vi "getWavelength_v80AM.vi"() -> ()   [LabVIEW 2016]
uses:
  x32/CLDevIFace.dll
panel:
  in  "Delay Time (s)":dbl=0.01
  out "XY Graph":cluster{i32[], dbl[]}(graph)
  out "error out":errorcluster
  out "output param":i32
  in  "stop":bool
  in  "OK Button":bool
  out "Wavelength":dbl format="%.9f"
  in  "CommPort":dbl=5.0 caption="Comm Port #"
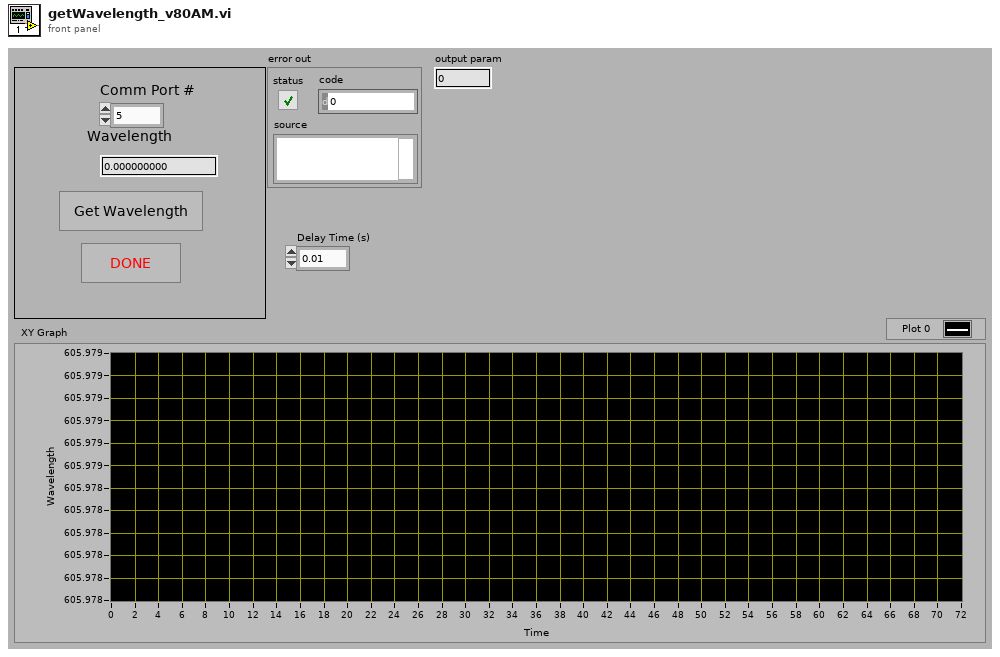
[diagram p1: front panel]
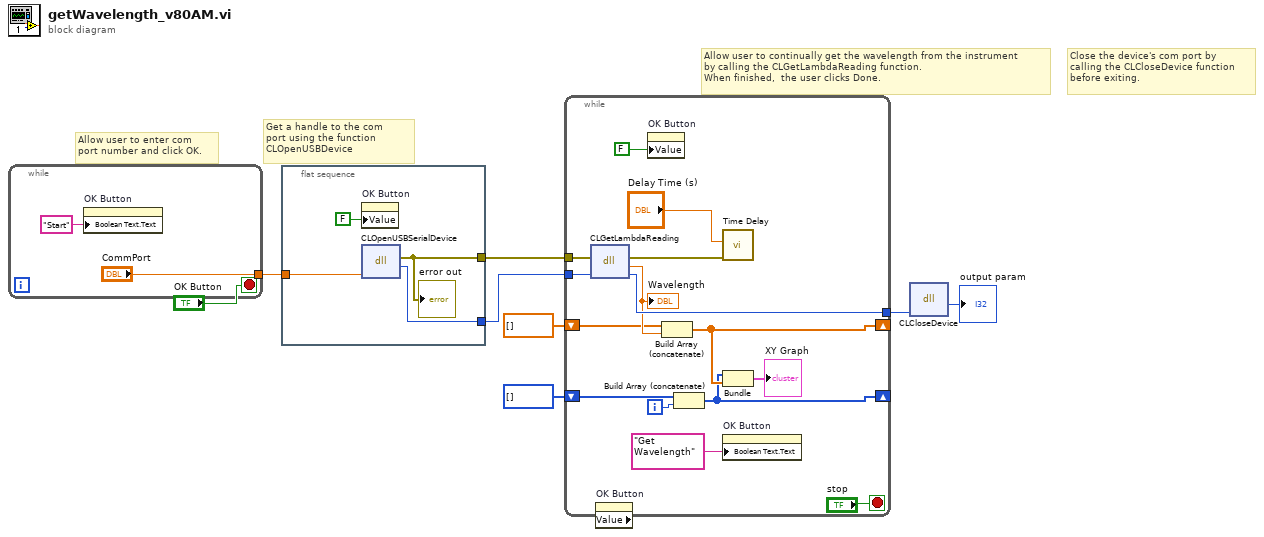
[diagram p0: block diagram]
diagram:
  # "Close the device's com port by\ncalling the CLCloseDevice function\nbefore exiting."
  # "Allow user to continually get the wavelength from the instrument\nby calling the CLGetLambdaReading function.  \nWhen finished,  the user clicks Done."
  # "Get a handle to the com\nport using the function CLOpenUSBDevice"
  # "Allow user to enter com \nport number and click OK."
  n1 = while {
    tunnel: ["CommPort"] -> w7
    stop <- "OK Button" stop-if-true
    n2 = property on="OK Button" class="Bool (strict)"("Boolean Text.Text"="Start") -> ()  [unwired: 2 in, 2 out]
  }
  n3 = flat-sequence {
    tunnel: w7 -> [w14]
    tunnel: [w13] -> w6
    tunnel: [w11] -> w1
    frame #0 {
      n4 = property on="OK Button" class="Bool (strict)"("Value"=FALSE) -> ()  [unwired: 2 in, 2 out]
      n5 = dll-call lib="C:/Users/Lab/Desktop/Bristol wavemeter 621/00424-2-00 621 customer CD/Programming Interface/x32/CLDevIface.dll" fn="CLOpenUSBSerialDevice"("commPort"=w14) -> (error out=w11:errorcluster, "return type"=w13:i32)  [unwired: 4 in, 1 out]
      "error out" <- w11
    }
  }
  n6 = while {
    tunnel: w6 -> [w29]
    tunnel: [w26] -> w5
    shift-right: [w20] -> _
    shift-left: dbl[] [] -> [w23]
    shift-right: [w19] -> _
    shift-left: i32[] [] -> [w22]
    tunnel: w1 -> [w15]
    i -> [w25]
    stop <- "stop" stop-if-true
    n7 = dll-call lib="C:/Users/Lab/Desktop/Bristol wavemeter 621/00424-2-00 621 customer CD/Programming Interface/x32/CLDevIface.dll" fn="CLGetLambdaReading"(error in=w15, "devHandle"=w29) -> (error out=w16:errorcluster, "return type"=w24:dbl, "devHandle"=w26:i32)  [unwired: 2 in, 1 out]
    "Wavelength" <- w24
    n8 = property on="OK Button" class="Bool (strict)" props=["Value"]() -> ()  [unwired: 2 in, 3 out]
    n9 = property on="OK Button" class="Bool (strict)"("Value"=FALSE) -> ()  [unwired: 2 in, 2 out]
    n10 = Build Array (concatenate)(w23, w24) -> (w20:dbl[])
    n11 = Build Array (concatenate)(w22, w25) -> (w19:i32[])
    n12 = call "Time Delay"("error in (no error)"=w16, "Delay Time (s)"="Delay Time (s)") -> ()  [unwired: 9 in, 1 out]
    n13 = Bundle(w19, w20) -> (→"XY Graph":cluster{i32[], dbl[]})  [unwired: 1 in]
    n14 = property on="OK Button" class="Bool (strict)"("Boolean Text.Text"="Get Wavelength") -> ()  [unwired: 2 in, 2 out]
  }
  n15 = dll-call lib="C:/Users/Lab/Desktop/Bristol wavemeter 621/00424-2-00 621 customer CD/Programming Interface/x32/CLDevIface.dll" fn="CLCloseDevice"("commPort"=w5) -> ("return type"=→"output param":i32)  [unwired: 4 in, 2 out]
